vi "Unbundle.vi"() -> ()   [LabVIEW 2020]
panel:
  out "Gender":bool
  out "Salary":u32
  out "Age":u8
  out "Name":string
  in  "employee":T1={"Name"="Atul Ghumade", "Age"=29, "Salary"=100000, "Gender"=TRUE}
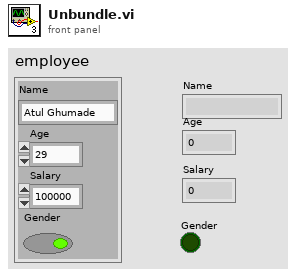
[diagram p1: front panel]
types:
  T1 = cluster{"Name":string, "Age":u8, "Salary":u32, "Gender":bool}
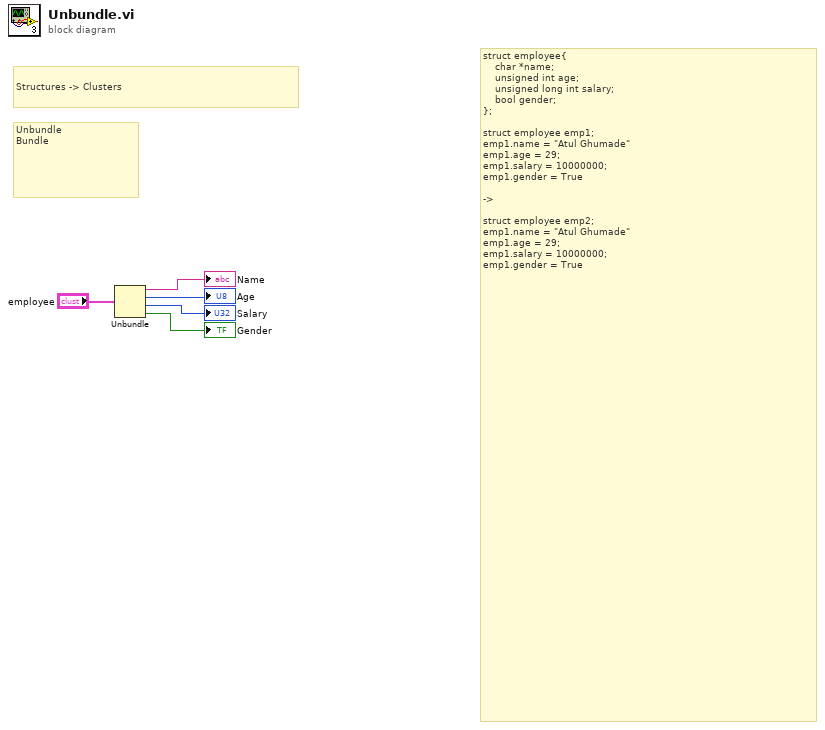
[diagram p0: block diagram]
diagram:
  # "Unbundle\nBundle"
  # "Structures -> Clusters"
  # "struct employee{\n    char *name;\n    unsigned int age;\n    unsigned long int salary;\n    bool gender;\n};\n\nstruct employee emp1;\nemp1.name = \"Atul Ghumade\"\nemp1.age = 29;\nemp1.salary = 10000000;\nemp1.gender = True\n\n->\n\nstruct employee emp2;\nemp1.name = \"Atul Ghumade\"\nemp1.age = 29;\nemp1.salary = 10000000;\nemp1.gender = True"
  n1 = Unbundle("employee") -> ("Name"=→"Name":string, "Age"=→"Age":u8, "Salary"=→"Salary":u32, "Gender"=→"Gender":bool)
